vi "Replot.vi"(8 "error in (no error)":errorcluster, 11 "Plot in":refnum<class "Plot.lvclass">) -> (0 "error out":errorcluster, 3 "Plot out":refnum<class "Plot.lvclass">)   [LabVIEW 2019, in "Plot.lvclass"]
uses:
  Plot.lvclass
  C:/Program Files/National Instruments/LabVIEW 2019/vi.lib/ActorFramework/Actor/Actor.lvclass
  Plot.lvclass/Plot.ctl
  <vilib>/ActorFramework/Actor/Actor.lvclass/Actor.ctl
  <vilib>/ActorFramework/Message Enqueuer/Message Enqueuer.lvclass/Message Enqueuer.ctl
  Write Replot request.vi
  Read Replot request.vi
  <vilib>/ActorFramework/Message Enqueuer/Init from Existing Queue.vi
  <vilib>/ActorFramework/Message Enqueuer/Enqueue.vi
  Plot Messages/Actual Replot Msg/Actual Replot Msg.lvclass
  C:/Program Files/National Instruments/LabVIEW 2019/vi.lib/ActorFramework/Message/Message.lvclass
  <vilib>/ActorFramework/Message Priority Queue/Priority Enqueue.vi
  <vilib>/ActorFramework/Message Enqueuer/Message Enqueuer.lvclass
  <vilib>/ActorFramework/Actor/Actor.lvclass
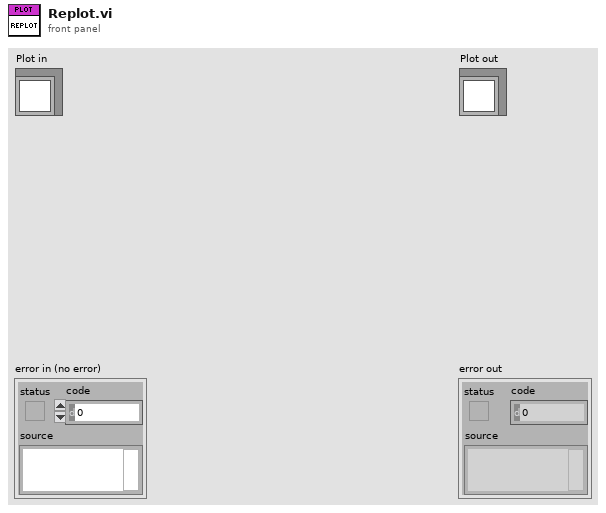
[diagram p1: front panel]
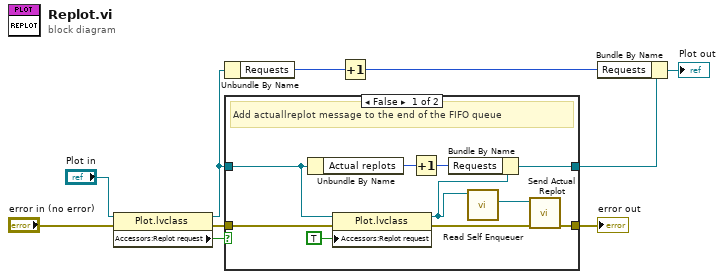
[diagram p0: block diagram]
diagram:
  n1 = property class="Plot.lvclass"(reference="Plot in", error in="error in (no error)") -> (reference out=w5:refnum<class "Plot.lvclass">, error out=w7:errorcluster, "Accessors:Replot request"=w8:bool)
  n2 = Unbundle By Name(w5) -> ("Requests"=w3:u64)
  n3 = case shown="False" w8 {
    tunnel: w5 -> [w16 w22]
    tunnel: w7 -> [w19 w21]
    tunnel: [w15 w22] -> w6
    tunnel: [w11 w21] -> w1
    frame False {
      # "Add actuallreplot message to the end of the FIFO queue"
      n4 = Unbundle By Name(w16) -> ("Actual replots"=w17:u64)
      n5 = property class="Plot.lvclass"(reference=w16, error in=w19, "Accessors:Replot request"=TRUE ("Replot request")) -> (reference out=w13:refnum<class "Plot.lvclass">, error out=w12:errorcluster)
      n6 = Increment(x=w17) -> (x+1=w18:u64)
      n7 = Bundle By Name(cluster=w13, "Requests"=w18) -> (w15:refnum<class "Plot.lvclass">)
      n8 = call <vilib>:"Read Self Enqueuer.vi"("Actor"=w13) -> ("Self Enqueuer"=w14:refnum<class "Message Enqueuer.lvclass">)  [unwired: 10 in]
      n9 = call "Send Actual Replot.vi"("error in (no error)"=w12, "Message Enqueuer"=w14) -> ("error out"=w11:errorcluster)  [unwired: 8 in, 1 out]
    }
    frame True {
      # "Already requested, ignore this message"
    }
  }
  "error out" <- w1
  n10 = Increment(x=w3) -> (x+1=w2:u64)
  n11 = Bundle By Name(cluster=w6, "Requests"=w2) -> (→"Plot out":refnum<class "Plot.lvclass">)
